vi "Try Match Abort.vi"(8 "error in":errorcluster, 10 "Data":u8[](array[numeric]), 11 "SDO Transfer in":refnum<class "SDO Transfer.lvclass">) -> (0 "error out":errorcluster, 2 "Match Found":bool, 3 "SDO Transfer out":refnum<class "SDO Transfer.lvclass">)   [LabVIEW 2020, in "SDO Manager.lvlib" / "SDO Transfer.lvclass"]
uses:
  SDO Transfer/SDO Transfer.lvclass
  SDO Transfer/SDO Transfer.lvclass/SDO Transfer.ctl
  SDO Transfer/SDO abort code.ctl
  Typedefs/SDO Result.ctl
  CANopen.lvlib
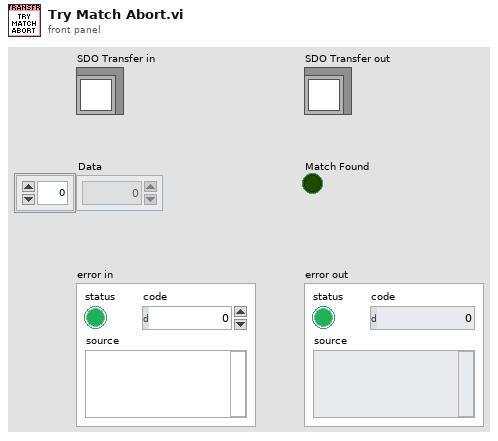
[diagram p1: front panel]
types:
  T1 = typedef "CANopen.lvlib/SDO Result.ctl" = cluster{"Success":bool, "SDO abort code":cluster{"Null":bool, "Value":T2}, "Data":cluster{"Null":bool, "Data":u8[]}}
  T2 = typedef "SDO Manager.lvlib/SDO Transfer.lvclass/SDO abort code.ctl" = u32
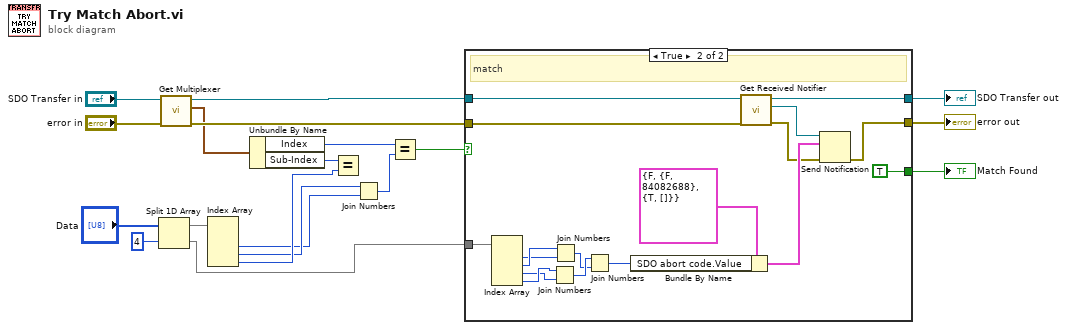
[diagram p0: block diagram]
diagram:
  n1 = Split 1D Array(array="Data", index=4) -> (first subarray=w6:u8[], second subarray=w4:u8[])
  n2 = call "Get Multiplexer.vi"("error in"="error in", "SDO Transfer in"="SDO Transfer in") -> ("error out"=w11:errorcluster, "Multiplexer"=w8:cluster{"Index":u16, "Sub-Index":u8}, "SDO Transfer out"=w9:refnum<class "SDO Transfer.lvclass">)  [unwired: 7 in]
  n3 = Index Array(array=w6) -> (element #2=w1:u8, element #3=w2:u8, element #4=w3:u8)  [unwired: 4 in, 1 out]
  n4 = Unbundle By Name(w8) -> ("Index"=w16:u16, "Sub-Index"=w17:u8)
  n5 = Equal?(x=w17, y=w3) -> ()  [unwired: 1 out]
  n6 = Join Numbers(hi=w2, lo=w1) -> ((hi.lo)=w18:u16)
  n7 = Equal?(x=w16, y=w18) -> (x = y?=w19:bool)
  n8 = case shown="True" w19 {
    tunnel: w11 -> [w21 w36]
    tunnel: w9 -> [w20 w35]
    tunnel: [w20 w33] -> w13
    tunnel: [w21 w28] -> w14
    tunnel: [_ TRUE] -> w15
    tunnel: w4 -> [_ w26]
    frame False {
      # "no match"
    }
    frame True {
      # "match"
      n9 = Index Array(array=w26) -> (element #1=w22:u8, element #2=w23:u8, element #3=w24:u8, element #4=w25:u8)  [unwired: 4 in]
      n10 = Join Numbers(hi=w25, lo=w24) -> ((hi.lo)=w38:u16)
      n11 = Join Numbers(hi=w23, lo=w22) -> ((hi.lo)=w37:u16)
      n12 = Join Numbers(hi=w38, lo=w37) -> ((hi.lo)=w31:u32)
      n13 = Bundle By Name(cluster=T1 {"Success"=FALSE, "SDO abort code"={"Null"=FALSE, "Value"=84082688}, "Data"={"Null"=TRUE, "Data"=[]}} ("notification"), "SDO abort code.Value"=w31) -> (w32:T1)
      n14 = call "Get Received Notifier.vi"("error in"=w36, "SDO Transfer in"=w35) -> ("error out"=w29:errorcluster, "Received Notifier"=w34:refnum<notifier>, "SDO Transfer out"=w33:refnum<class "SDO Transfer.lvclass">)  [unwired: 7 in]
      n15 = Send Notification(notification=w32, notifier=w34, error in (no error)=w29) -> (error out=w28:errorcluster)  [unwired: 1 out]
    }
  }
  "Match Found" <- w15
  "error out" <- w14
  "SDO Transfer out" <- w13
